vi "Read Osc. Energy Density.vi"(0 "object in":refnum<class "TBS2000Series.lvclass">, 7 "Oscilloscope":T2={"Source Prefocus"=2, "Source Main"=2, "Source Probe"=1} {"Source Probe" items=["Math", "Channel 1", "Channel 2", "Channel 3", "Channel 4"]; "Source Main" items=["Math", "Channel 1", "Channel 2", "Channel 3", "Channel 4"]; "Source Prefocus" items=["Math", "Channel 1", "Channel 2", "Channel 3", "Channel 4"]}, 11 "error in (no error)":errorcluster) -> (4 "object out":refnum<class "TBS2000Series.lvclass">, 8 "Oscilloscope\n Results":T1 {"Probe Current" format="%.2p"; "Phase Angle" format="%.2p"; "Main Freq" format="%.2p"; "Main Volt" format="%.2p"; "Prefocus Freq" format="%.2p"; "Prefocus Volt" format="%.2p"}, 15 "error out":errorcluster)   [LabVIEW 2023, in "TBS2000Series.lvclass"]
uses:
  TBS2000Series.lvclass
  TBS2000Series.lvclass/TBS2000Series.ctl
  <instrlib>/Tektronix TBS 2000 Series/Tektronix TBS 2000 Series.lvlib
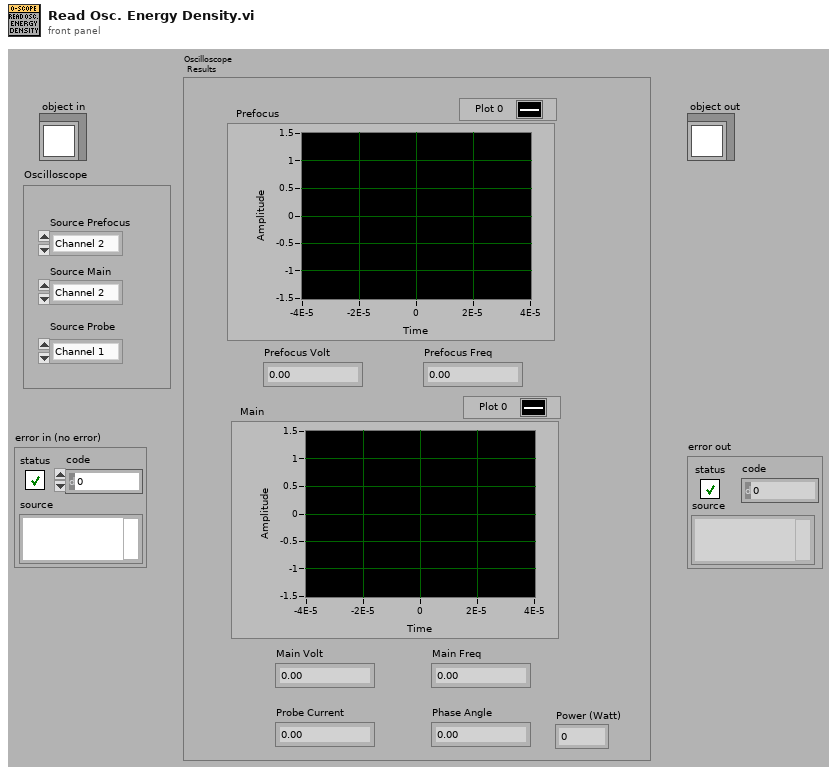
[diagram p1: front panel]
types:
  T1 = cluster{"Prefocus":cluster{"Initial X":dbl, "X Increment":dbl, "Waveform Array":dbl[]}, "Prefocus Volt":dbl, "Prefocus Freq":dbl, "Main":cluster{"Initial X":dbl, "X Increment":dbl, "Waveform Array":dbl[]}, "Main Volt":dbl, "Main Freq":dbl, "Phase Angle":dbl, "Probe Current":dbl, "Power (Watt)":dbl}
  T2 = cluster{"Source Prefocus":i32, "Source Main":i32, "Source Probe":i32}
  T3 = cluster{"Initial X":dbl, "X Increment":dbl, "Waveform Array":dbl[]}
  T4 = cluster{"Waveform Graph":cluster{"Initial X":dbl, "X Increment":dbl, "Waveform Array":dbl[]}, "Measurement":dbl, "Measurement":dbl, "Waveform Graph":cluster{"Initial X":dbl, "X Increment":dbl, "Waveform Array":dbl[]}, "Measurement":dbl, "Measurement":dbl, "Measurement":dbl, dbl, dbl}
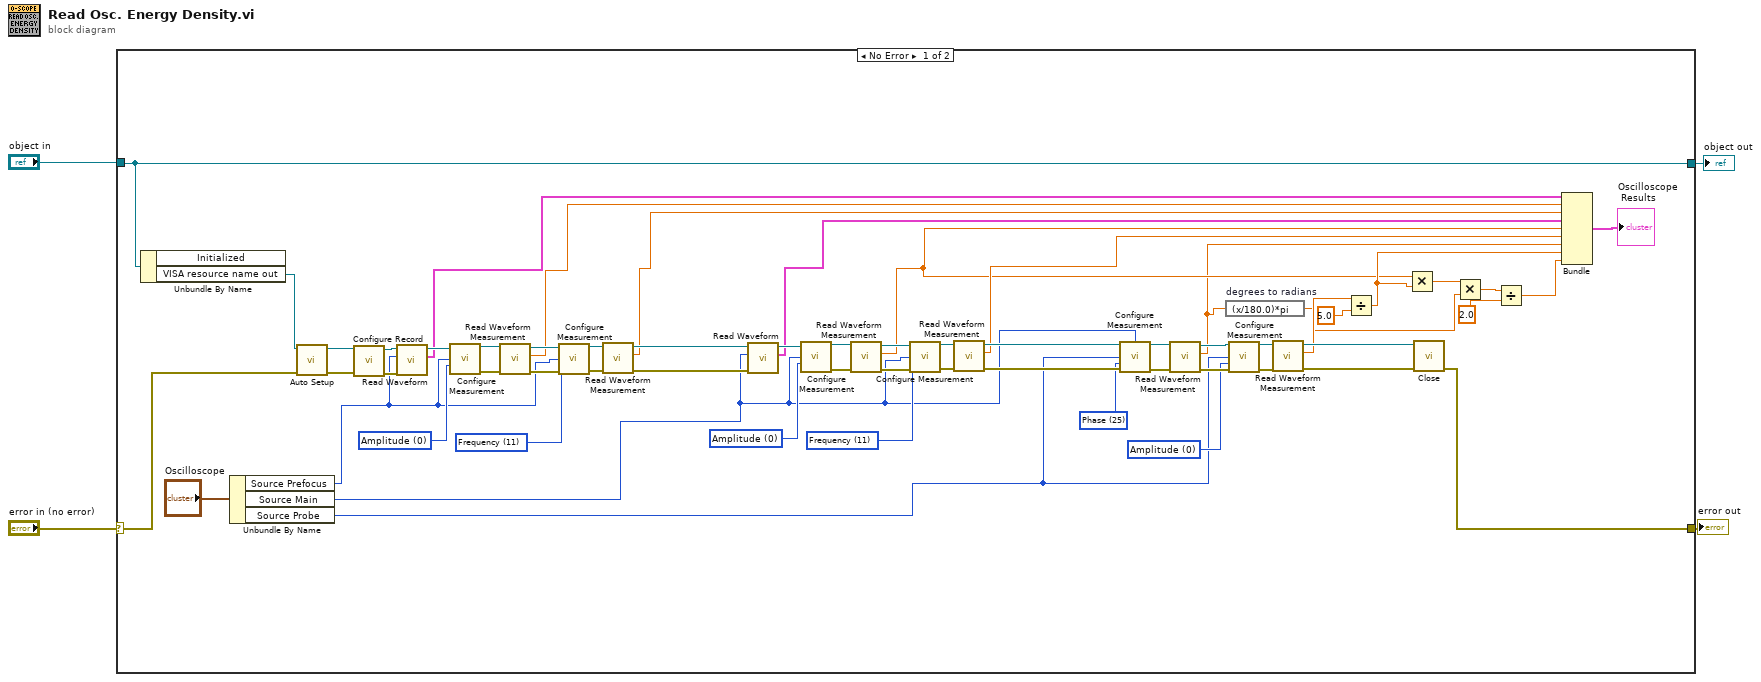
[diagram p0: block diagram]
diagram:
  n1 = case shown="No Error" "error in (no error)" {
    selector: "error in (no error)" -> [w50 w66]
    tunnel: [w49 w66] -> w3
    tunnel: [w51 w65] -> w1
    tunnel: "object in" -> [w51 w65]
    frame No Error {
      w26 = 0 items=["Amplitude", "Area", "Burst", "Cycle Area", "Cycle Mean", "Cycle RMS", "Delay RR", "Delay RF", "Delay FR", "Delay FF", "Fall Time", "Frequency", "High Reference", "Low Reference", "Max", "Mean", "Min", "- Duty Cycle", "- Edge Count", "- Overshoot", "- Pulse Count", "- Width", "+ Duty Cycle", "+ Edge Count", "Period", "Phase", "Peak-to-Peak", "+ Overshoot", "+ Pulse Count", "+ Width", "Rise", "RMS"] ("Measurement Type (30: Rise)")
      w27 = 25 items=["Amplitude", "Area", "Burst", "Cycle Area", "Cycle Mean", "Cycle RMS", "Delay RR", "Delay RF", "Delay FR", "Delay FF", "Fall Time", "Frequency", "High Reference", "Low Reference", "Max", "Mean", "Min", "- Duty Cycle", "- Edge Count", "- Overshoot", "- Pulse Count", "- Width", "+ Duty Cycle", "+ Edge Count", "Period", "Phase", "Peak-to-Peak", "+ Overshoot", "+ Pulse Count", "+ Width", "Rise", "RMS"] ("Measurement Type (30: Rise)")
      w41 = 11 items=["Amplitude", "Area", "Burst", "Cycle Area", "Cycle Mean", "Cycle RMS", "Delay RR", "Delay RF", "Delay FR", "Delay FF", "Fall Time", "Frequency", "High Reference", "Low Reference", "Max", "Mean", "Min", "- Duty Cycle", "- Edge Count", "- Overshoot", "- Pulse Count", "- Width", "+ Duty Cycle", "+ Edge Count", "Period", "Phase", "Peak-to-Peak", "+ Overshoot", "+ Pulse Count", "+ Width", "Rise", "RMS"] ("Measurement Type (30: Rise)")
      w48 = 0 items=["Amplitude", "Area", "Burst", "Cycle Area", "Cycle Mean", "Cycle RMS", "Delay RR", "Delay RF", "Delay FR", "Delay FF", "Fall Time", "Frequency", "High Reference", "Low Reference", "Max", "Mean", "Min", "- Duty Cycle", "- Edge Count", "- Overshoot", "- Pulse Count", "- Width", "+ Duty Cycle", "+ Edge Count", "Period", "Phase", "Peak-to-Peak", "+ Overshoot", "+ Pulse Count", "+ Width", "Rise", "RMS"] ("Measurement Type (0: Amplitude)")
      w53 = 11 items=["Amplitude", "Area", "Burst", "Cycle Area", "Cycle Mean", "Cycle RMS", "Delay RR", "Delay RF", "Delay FR", "Delay FF", "Fall Time", "Frequency", "High Reference", "Low Reference", "Max", "Mean", "Min", "- Duty Cycle", "- Edge Count", "- Overshoot", "- Pulse Count", "- Width", "+ Duty Cycle", "+ Edge Count", "Period", "Phase", "Peak-to-Peak", "+ Overshoot", "+ Pulse Count", "+ Width", "Rise", "RMS"] ("Measurement Type (30: Rise)")
      w60 = 0 items=["Amplitude", "Area", "Burst", "Cycle Area", "Cycle Mean", "Cycle RMS", "Delay RR", "Delay RF", "Delay FR", "Delay FF", "Fall Time", "Frequency", "High Reference", "Low Reference", "Max", "Mean", "Min", "- Duty Cycle", "- Edge Count", "- Overshoot", "- Pulse Count", "- Width", "+ Duty Cycle", "+ Edge Count", "Period", "Phase", "Peak-to-Peak", "+ Overshoot", "+ Pulse Count", "+ Width", "Rise", "RMS"] ("Measurement Type (0: Amplitude)")
      n2 = Unbundle By Name(w51) -> ("VISA resource name out"=w23:refnum<visa-resource-name>)  [unwired: 1 out]
      n3 = Unbundle By Name("Oscilloscope") -> ("Source Prefocus"=w21:i32, "Source Main"=w20:i32, "Source Probe"=w19:i32)
      n4 = call <instrlib>:"Auto Setup.vi"("error in (no error)"=w50, "VISA resource name"=w23) -> ("error out"=w63:errorcluster, "VISA resource name out"=w64:refnum<visa-resource-name>)  [unwired: 8 in]
      n5 = call <instrlib>:"Configure Record.vi"("error in (no error)"=w63, "VISA resource name"=w64) -> ("error out"=w61:errorcluster, "VISA resource name out"=w62:refnum<visa-resource-name>)  [unwired: 8 in]
      n6 = call <instrlib>:"Read Waveform.vi"("error in (no error)"=w61, "Source (1: Channel 1)"=w21, "VISA resource name"=w62) -> ("Waveform Graph"=w17:T3, "VISA resource name out"=w52:refnum<visa-resource-name>)  [unwired: 6 in, 1 out]
      n7 = call <instrlib>:"Configure Measurement.vi"("VISA resource name"=w52, "Measurement Source 1 (1: Channel 1)"=w21, "Measurement Type (30: Rise)"=w60) -> ("VISA resource name out"=w59:refnum<visa-resource-name>, "error out"=w58:errorcluster)  [unwired: 11 in]
      n8 = call <instrlib>:"Read Waveform Measurement.vi"("error in (no error)"=w58, "VISA resource name"=w59) -> ("error out"=w54:errorcluster, "Measurement"=w16:dbl, "VISA resource name out"=w56:refnum<visa-resource-name>)  [unwired: 7 in]
      n9 = call <instrlib>:"Configure Measurement.vi"("VISA resource name"=w56, "Measurement Source 1 (1: Channel 1)"=w21, "Measurement Type (30: Rise)"=w53, "error in (no error)"=w54) -> ("VISA resource name out"=w57:refnum<visa-resource-name>, "error out"=w55:errorcluster)  [unwired: 10 in]
      n10 = call <instrlib>:"Read Waveform Measurement.vi"("error in (no error)"=w55, "VISA resource name"=w57) -> ("error out"=w38:errorcluster, "Measurement"=w15:dbl, "VISA resource name out"=w39:refnum<visa-resource-name>)  [unwired: 7 in]
      n11 = call <instrlib>:"Read Waveform.vi"("error in (no error)"=w38, "Source (1: Channel 1)"=w20, "VISA resource name"=w39) -> ("Waveform Graph"=w14:T3, "VISA resource name out"=w40:refnum<visa-resource-name>)  [unwired: 6 in, 1 out]
      n12 = call <instrlib>:"Configure Measurement.vi"("VISA resource name"=w40, "Measurement Source 1 (1: Channel 1)"=w20, "Measurement Type (30: Rise)"=w48) -> ("VISA resource name out"=w47:refnum<visa-resource-name>, "error out"=w46:errorcluster)  [unwired: 11 in]
      n13 = call <instrlib>:"Read Waveform Measurement.vi"("error in (no error)"=w46, "VISA resource name"=w47) -> ("error out"=w42:errorcluster, "Measurement"=w7:dbl, "VISA resource name out"=w44:refnum<visa-resource-name>)  [unwired: 7 in]
      n14 = call <instrlib>:"Configure Measurement.vi"("VISA resource name"=w44, "Measurement Source 1 (1: Channel 1)"=w20, "Measurement Type (30: Rise)"=w41, "error in (no error)"=w42) -> ("VISA resource name out"=w45:refnum<visa-resource-name>, "error out"=w43:errorcluster)  [unwired: 10 in]
      n15 = call <instrlib>:"Read Waveform Measurement.vi"("error in (no error)"=w43, "VISA resource name"=w45) -> ("error out"=w32:errorcluster, "Measurement"=w13:dbl, "VISA resource name out"=w37:refnum<visa-resource-name>)  [unwired: 7 in]
      n16 = call <instrlib>:"Configure Measurement.vi"("VISA resource name"=w37, "Measurement Source 2 (2: Channel 2)"=w20, "Measurement Source 1 (1: Channel 1)"=w19, "Measurement Type (30: Rise)"=w27, "error in (no error)"=w32) -> ("VISA resource name out"=w36:refnum<visa-resource-name>, "error out"=w31:errorcluster)  [unwired: 9 in]
      n17 = call <instrlib>:"Read Waveform Measurement.vi"("error in (no error)"=w31, "VISA resource name"=w36) -> ("error out"=w30:errorcluster, "Measurement"=w6:dbl, "VISA resource name out"=w35:refnum<visa-resource-name>)  [unwired: 7 in]
      n18 = expression code="(x/180.0)*pi" "degrees to radians"(w6) -> (w5:dbl)
      n19 = call <instrlib>:"Configure Measurement.vi"("VISA resource name"=w35, "Measurement Source 1 (1: Channel 1)"=w19, "Measurement Type (30: Rise)"=w26, "error in (no error)"=w30) -> ("VISA resource name out"=w34:refnum<visa-resource-name>, "error out"=w29:errorcluster)  [unwired: 10 in]
      n20 = call <instrlib>:"Read Waveform Measurement.vi"("error in (no error)"=w29, "VISA resource name"=w34) -> ("error out"=w28:errorcluster, "Measurement"=w25:dbl, "VISA resource name out"=w33:refnum<visa-resource-name>)  [unwired: 7 in]
      n21 = Divide(x=w25, y=5.0) -> (x/y=w8:dbl)
      n22 = Multiply(x=w7, y=w8) -> (x*y=w9:dbl)
      n23 = call <instrlib>:"Close.vi"("error in (no error)"=w28, "VISA resource name"=w33) -> ("error out"=w49:errorcluster)  [unwired: 9 in]
      n24 = Multiply(x=w9, y=w5) -> (x*y=w12:dbl)
      n25 = Divide(x=w12, y=2.0) -> (x/y=w10:dbl)
      n26 = Bundle("Waveform Graph"=w17, "Measurement"=w16, "Measurement"=w15, "Waveform Graph"=w14, "Measurement"=w7, "Measurement"=w13, "Measurement"=w6, w8, w10) -> (→"Oscilloscope\n Results":T4)  [unwired: 1 in]
    }
    frame Error {
    }
  }
  "error out" <- w3
  "object out" <- w1
